vi "sv_Flat Pink Filter (DBL).vi"(6 "unity gain freq (rad/s)":dbl=1.0 format="%.2g", 7 "reset":bool, 9 "lower cutoff freq":dbl=0.1, 10 "fs":dbl=1000.0 format="%.2f", 11 "X":dbl[](array[numeric])) -> (0 "error":i32, 1 "magnitude error (dB)":T2, 2 "filter information":T1, 3 "Filtered X":dbl[](array[numeric]), 4 "noise bandwidth":dbl=1.0 format="%.2g")   [LabVIEW 2017]
uses:
  <vilib>/Analysis/baseanly.llb/IIR Cascade Filter (DBL).vi
  <vilib>/Analysis/NI_AALBase.lvlib
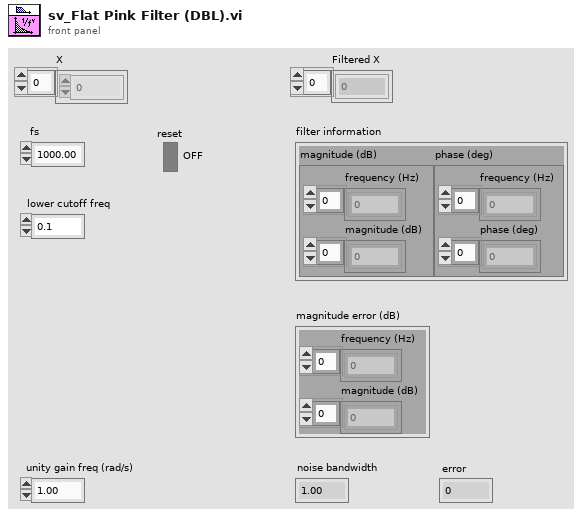
[diagram p1: front panel]
types:
  T1 = cluster{"magnitude (dB)":cluster{"frequency (Hz)":dbl[], "magnitude (dB)":dbl[]}, "phase (deg)":cluster{"frequency (Hz)":dbl[], "phase (deg)":dbl[]}}
  T2 = cluster{"frequency (Hz)":dbl[], "magnitude (dB)":dbl[]}
  T3 = cluster{"filter structure":enum32{"IIR 2nd Order", "IIR 4th Order"}, "Reverse Coefficients":dbl[], "Forward Coefficients":dbl[]}
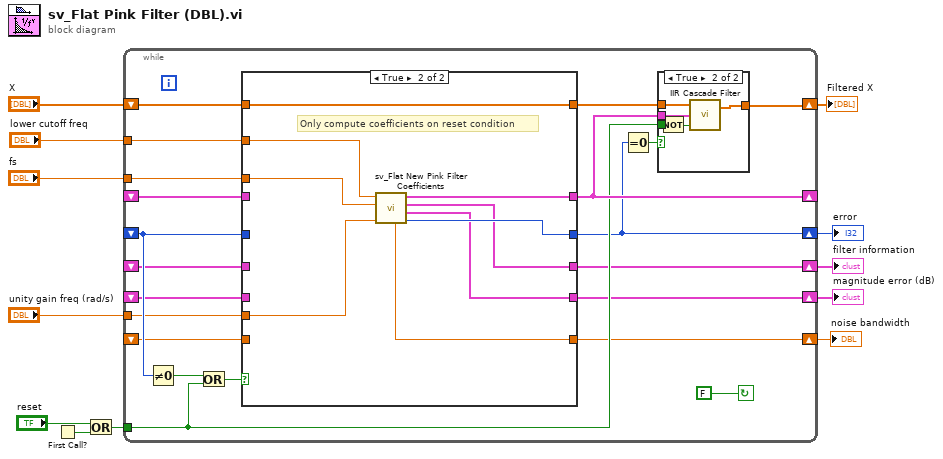
[diagram p0: block diagram]
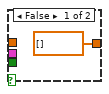
[diagram p2: hidden frame]
diagram:
  n1 = First Call?() -> (First Call?: T/F=w7:bool)
  n2 = Or(x="reset", y=w7) -> (x .or. y?=w8:bool)
  n3 = while {
    tunnel: w8 -> [w25]
    shift-left: _ -> [w31]
    shift-right: [w32] -> _
    tunnel: "fs" -> [w28]
    shift-right: [w23] -> w5
    shift-left: _ -> [w26]
    shift-right: [w21] -> w11
    shift-left: _ -> [w20]
    shift-right: [w19] -> w12
    shift-left: _ -> [w18]
    tunnel: "unity gain freq (rad/s)" -> [w17]
    shift-right: [w16] -> w9
    shift-left: _ -> [w15]
    shift-right: [w14] -> w3
    shift-left: "X" -> [w30]
    tunnel: "lower cutoff freq" -> [w13]
    stop <- FALSE continue-if-true
    n4 = Not Equal To 0?(x=w26) -> (x != 0?=w27:bool)
    n5 = Or(x=w27, y=w25) -> (x .or. y?=w24:bool)
    n6 = case shown="True" w24 {
      tunnel: [w45 w53] -> w32
      tunnel: w31 -> [w45 _]
      tunnel: w30 -> [w44 w54]
      tunnel: [w44 w54] -> w29
      tunnel: w28 -> [_ w47]
      tunnel: [w43 w52] -> w23
      tunnel: w26 -> [w43 _]
      tunnel: [w42 w51] -> w21
      tunnel: w20 -> [w42 _]
      tunnel: [w41 w50] -> w19
      tunnel: w18 -> [w41 _]
      tunnel: w17 -> [_ w48]
      tunnel: [w40 w49] -> w16
      tunnel: w15 -> [w40 _]
      tunnel: w13 -> [_ w46]
      frame False {
      }
      frame True {
        # "Only compute coefficients on reset condition"
        n7 = call <vilib>:"sv_Flat New Pink Filter Coefficients.vi"("unity gain freq (rad/s)"=w48, "fs"=w47, "lower cutoff freq"=w46) -> ("error"=w52:i32, "magnitude error (dB)"=w50:T2, "filter information"=w51:T1, "IIR Filter Cluster"=w53:T3, "noise bandwidth"=w49:dbl)  [unwired: 4 in]
      }
    }
    n8 = Equal To 0?(x=w23) -> (x = 0?=w22:bool)
    n9 = case shown="True" w22 {
      tunnel: w32 -> [_ w39]
      tunnel: w29 -> [_ w38]
      tunnel: [dbl[] [] ("Filtered X") w37] -> w14
      tunnel: w25 -> [_ w35]
      frame False {
      }
      frame True {
        n10 = Not(x=w35) -> (.not. x?=w36:bool)
        n11 = call-poly <vilib>:"IIR Cascade Filter.vi"("init/cont (init:F)"=w36, "IIR Filter Cluster"=w39, "X"=w38) -> ("Filtered X"=w37:dbl[])  [unwired: 1 out]
      }
    }
  }
  "Filtered X" <- w3
  "error" <- w5
  "noise bandwidth" <- w9
  "filter information" <- w11
  "magnitude error (dB)" <- w12
